vi "Simulate Joysticks.vi"(10 "Send Inputs":bool, 11 "Joystick Inputs":T2(array[cluster])) -> (3 "Joystick Inputs":T1)   [LabVIEW 2025]
uses:
  swerve/Type Definitions/Data/Robot Velocities.ctl
  d4d6f690-fe6c-42a4-b1af-8ca75be83e18.vi
panel:
  out "Current Time":dbl
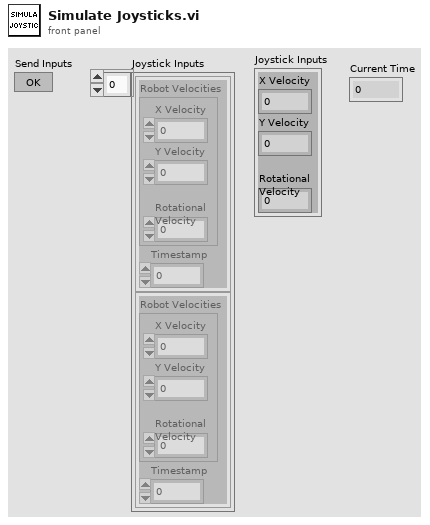
[diagram p1: front panel]
types:
  T1 = typedef "Robot Velocities.ctl" = cluster{"X Velocity":dbl, "Y Velocity":dbl, "Rotational \nVelocity":dbl}
  T2 = cluster{"Robot Velocities":T1, "Timestamp":dbl}[]
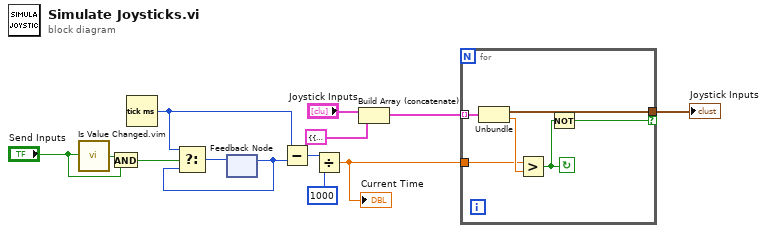
[diagram p0: block diagram]
diagram:
  n1 = call "Is Value Changed.vim"("value"="Send Inputs") -> ("changed or first call?"=w9:bool)
  n2 = And(x=w9, y="Send Inputs") -> (x .and. y?=w7:bool)
  n3 = Tick Count (ms)() -> (millisecond timer value=w4:u32)
  n4 = feedback #1() -> (w5:u32)  [unwired: 1 in]
  n5 = Select(t=w4, s=w7, f=w5) -> (s? t:f=w6:u32)
  n6 = feedback-in #1(w6) -> ()
  n7 = Subtract(x=w4, y=w5) -> (x-y=w3:u32)
  n8 = Divide(x=w3, y=u32 1000) -> (x/y=w1:dbl)
  "Current Time" <- w1
  n9 = Build Array (concatenate)("Joystick Inputs", cluster{"Robot Velocities":T1, "Timestamp":dbl} {"Robot Velocities"={"X Velocity"=0.0, "Y Velocity"=0.0, "Rotational \nVelocity"=0.0}, "Timestamp"=inf}) -> (w10:T2)
  n10 = for {
    tunnel: w10 -> [w19] mode=indexing
    tunnel: w1 -> [w16]
    tunnel: [w18] -> w13 if=w14
    stop <- w15 continue-if-true
    n11 = Unbundle(w19) -> ("Robot Velocities"=w18:T1, "Timestamp"=w17:dbl)
    n12 = Greater?(x=w16, y=w17) -> (0:w15:bool)
    n13 = Not(x=w15) -> (.not. x?=w14:bool)
  }
  "Joystick Inputs" <- w13
